vi "DigiComm_RX.vi"(7 "filter parameters":T1={"Alpha"=0.5, "Filter Length"=6, "TX Filter"=enum."Root Raised Cos"} {"Alpha" format="%.2f"}, 8 "Number of Symbols":i32=100, 9 "Mapping Parameters":T2={"Modulation Order (M)"=2, "Modulation Type"=0, "Samples per Symbol"=8} {"Modulation Type" items=["PSK", "QAM"]}, 10 "data waveform":T3={"t0"=0.0, "dt"=1.0, "Y"=[]} {"Y" format="%.3f"; "dt" format="%^.2e"; "t0" format="%.4f"}) -> (2 "Output Bit Stream":i8[](array[numeric]))   [LabVIEW 2011]
uses:
  <vilib>/addons/Modulation/Analog/controls/Complex Data Waveform.ctl
  subVIs_Dcomm_offered/FilterCoefficient.ctl
  <vilib>/addons/Modulation/niDMT.lvlib
  <vilib>/addons/Modulation/niAMT.lvlib
panel:
  out "RX matched filter":dbl[](graph)
  out "Constellation Graph":T4(graph)
  in  "autoscale":bool
  # "Lab 2(b): Digital Communication (RX)"
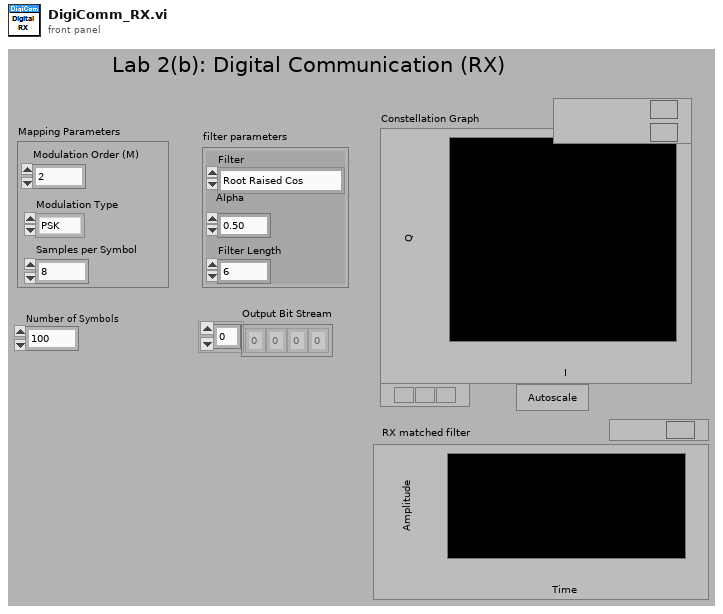
[diagram p1: front panel]
types:
  T1 = typedef "FilterCoefficient.ctl" = cluster{"Alpha":dbl, "Filter Length":i32, "TX Filter":enum16{"Root Raised Cos", "Raised Cos", "Rectangular"}}
  T2 = cluster{"Modulation Order (M)":i32, "Modulation Type":u16, "Samples per Symbol":i32}
  T3 = typedef "niAMT.lvlib/Complex Data Waveform.ctl" = cluster{"t0":dbl, "dt":dbl, "Y":cdb[]}
  T4 = cluster{"Decimated Array":dbl[], "Decimated Array":dbl[]}[]
  T5 = cluster{"samples per symbol (16)":i32, "symbol map":cdb[]}
  T6 = cluster{"constellation":dbl[], "oversampled data":dbl[]}[]
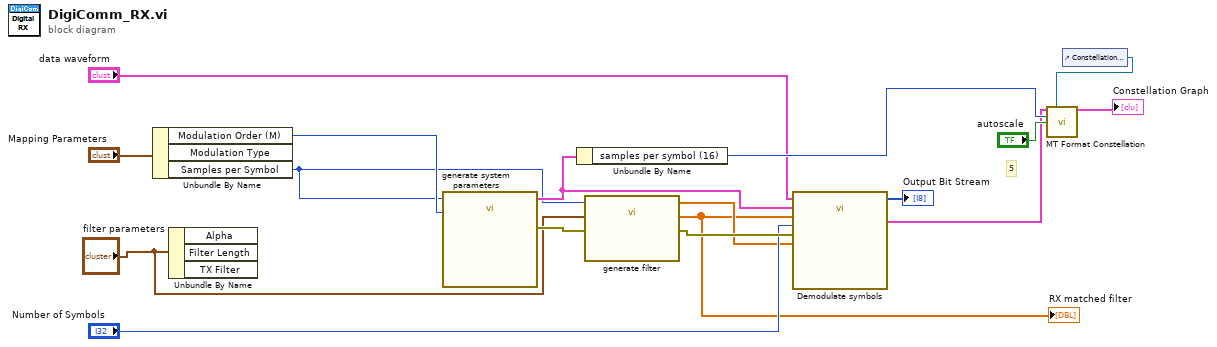
[diagram p0: block diagram]
diagram:
  # "5"
  n1 = Unbundle By Name("Mapping Parameters") -> ("Modulation Order (M)"=w9:i32, "Samples per Symbol"=w8:i32)  [unwired: 1 out]
  n2 = Unbundle By Name("filter parameters") -> ()  [unwired: 3 out]
  n3 = call "generate system parameters.vi"("M-PSK"=w9, "samples per symbol"=w8) -> ("error out"=w15:errorcluster, "system parameters"=w17:T5)  [unwired: 8 in]
  n4 = Unbundle By Name(w17) -> ("samples per symbol (16)"=w16:i32)
  n5 = call "generate filter.vi"("error in (no error)"=w15, "filter parameters"="filter parameters", "pulse shaping samples per symbol (16)"=w8) -> ("error out"=w11:errorcluster, "matched filter coefficients"=w1:dbl[], "pulse shaping filter coefficients"=w2:dbl[])  [unwired: 6 in]
  "RX matched filter" <- w1
  n6 = call "Demodulate symbols.vi"("input complex waveform"="data waveform", "PSK system parameters"=w17, "matched filter coefficients"=w1, "Number of Symbols"="Number of Symbols", "error in (no error)"=w11, "TX Pulse Shaping Filter Coefficients"=w2) -> ("Output Bit Stream"=→"Output Bit Stream":i8[], "output complex waveform"=w3:T3)  [unwired: 7 in, 1 out]
  n7 = control-ref of="Constellation Graph"() -> (w13:refnum<vi>)
  n8 = call <vilib>:"MT Format Constellation.vi"("waveform"=w3, "constellation reference"=w13, "samples per symbol"=w16, "autoscale"="autoscale") -> ("constellation graph"=→"Constellation Graph":T6)  [unwired: 10 in, 1 out]
